vi "LookUpHighRate.vi"(8 "error in (no error)":errorcluster, 10 "MetricDefinitionInstanceId":string, 11 "Metric Cache":variant) -> (0 "error out":errorcluster, 2 "high rate":bool, 3 "Metric Cache Out":variant)   [LabVIEW 2017, in "AnalysisHelper.lvlib"]
uses:
  <vilib>/addons/InsightCM/Utilities/Analysis/Shared/AnalysisHelper.lvlib
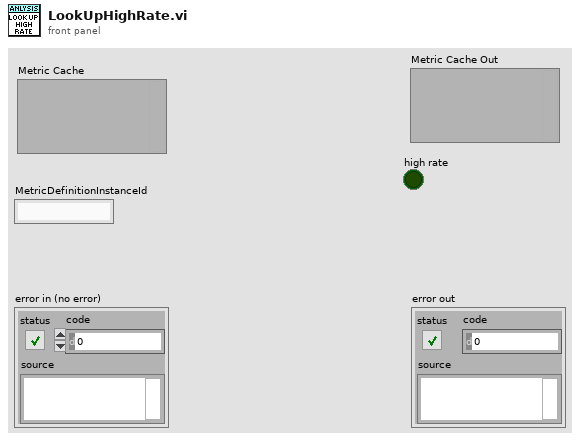
[diagram p1: front panel]
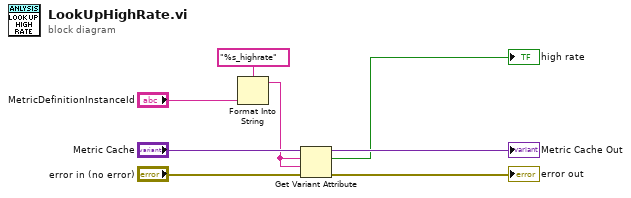
[diagram p0: block diagram]
diagram:
  n1 = Format Into String(format string="%s_highrate", "MetricDefinitionInstanceId") -> (resulting string=w1:string)  [unwired: 2 in, 1 out]
  n2 = Get Variant Attribute(Variant="Metric Cache", name=w1, default value (empty Variant)=w1, error in="error in (no error)") -> (duplicate Variant=→"Metric Cache Out":variant, found=→"high rate":bool, error out=→"error out":errorcluster)  [unwired: 1 out]
